vi "qIFC.vi"(0 "System no.":i32=1 min=1 step=1, 2 "Interface parameter":string[](array[string]), 3 "All Parameters?":bool, 5 "error in":errorcluster) -> (14 "Parameter value":string[](array[string]), 15 "interface parameter out":string[](array[string]), 19 "error out":errorcluster)   [LabVIEW 2026]
doc: "Returns the current interface configuration.\n\nE-517, E-518, E-753, E-754, E-871, E-872, E-873, E-874: Note that when the controller is part of a network with DHCP, the static IP address of the controller is returned, not the currently used IP address which was obtained from the DHCP server.\n\nF-206, M-8X0: Only for GCS syntax version = GCS 2.0 or higher (Check with CSV?.vi. If CSV?.vi is not supported, syntax version is GCS 1.0)."
panel:
  # "Returns the current interface configuration."
  # "Query"
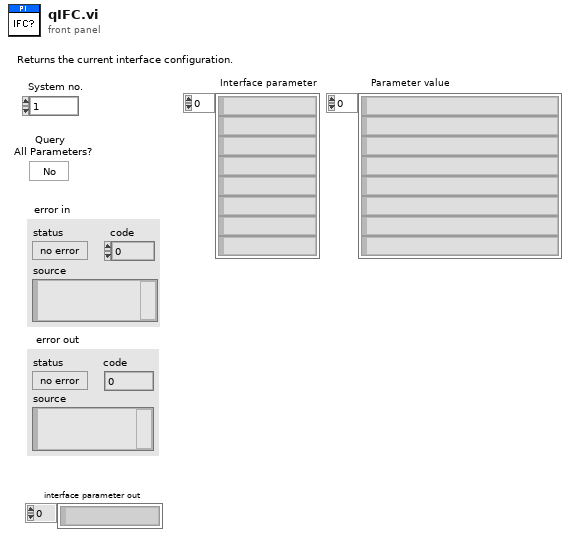
[diagram p1: front panel]
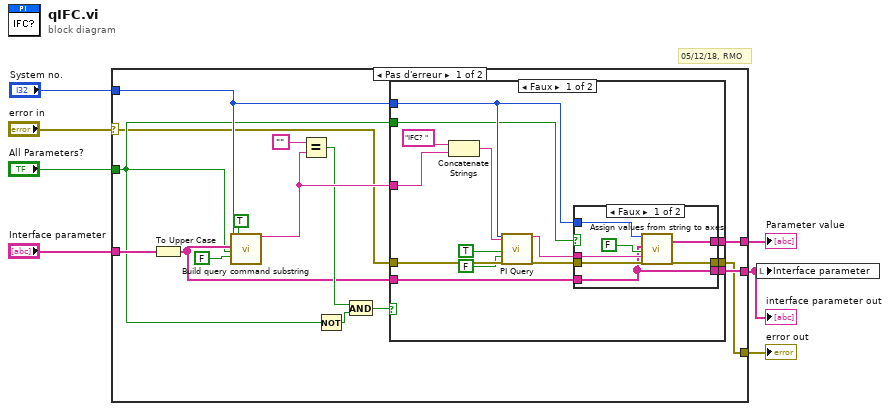
[diagram p0: block diagram]
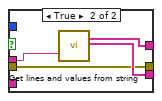
[diagram p2: hidden frame]
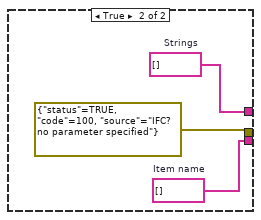
[diagram p3: hidden frame]
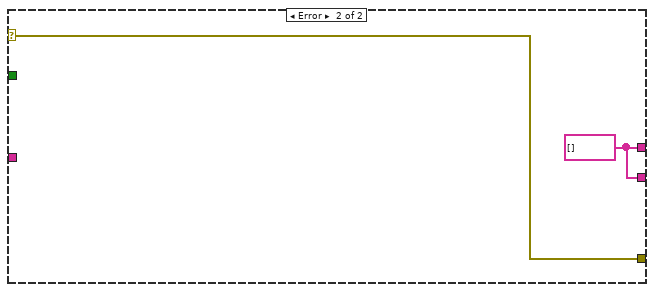
[diagram p4: hidden frame]
diagram:
  # "05/12/18, RMO"
  n1 = case shown="Pas d'erreur" "error in" {
    selector: "error in" -> [w10 w51]
    tunnel: "Interface parameter" -> [w22 _]
    tunnel: [w9 w51] -> w6
    tunnel: "System no." -> [w19 _]
    tunnel: "All Parameters?" -> [w13 _]
    tunnel: [w16 w52] -> w3
    tunnel: [w12 w52] -> w2
    frame No Error {
      n2 = To Upper Case(1:w22) -> (0:w14:string[])
      n3 = call "Build query command substring.vi"("System no."=w19, "Axes to query in"=w14, "Query\nAll axes?"=w13, "For all axes: use\nAxis identifier?"=FALSE ("For all axes: use\nAxis identifier?"), "With space?"=TRUE) -> ("Command substring"=w20:string)  [unwired: 1 in, 13 out]
      n4 = Equal?(x="", y=w20) -> (x = y?=w17:bool)
      n5 = Not(x=w13) -> (.not. x?=w18:bool)
      n6 = And(x=w17, y=w18) -> (x .and. y?=w8:bool)
      n7 = case shown="Faux" w8 {
        tunnel: w20 -> [w33 _]
        tunnel: w19 -> [w32 _]
        tunnel: [w31 w49] -> w16
        tunnel: w14 -> [w30 _]
        tunnel: w13 -> [w29 _]
        tunnel: [w28 w48] -> w12
        tunnel: w10 -> [w27 _]
        tunnel: [w23 errorcluster {"status"=TRUE, "code"=100, "source"="IFC? no parameter specified"} ("error out")] -> w9
        frame False {
          n8 = Concatenate Strings("IFC? ", w33) -> (w34:string)
          n9 = call "PI Query.vi"("System no."=w32, "String to send"=w34, "Attach termination char.?"=TRUE ("Attach Linefeed?"), "Strip spaces?"=FALSE, "error in"=w27) -> ("String read"=w25:string, "error out"=w24:errorcluster)  [unwired: 2 in, 11 out]
          n10 = case shown="Faux" w29 {
            tunnel: w32 -> [w43 _]
            tunnel: w25 -> [w42 w47]
            tunnel: [w41 w46] -> w31
            tunnel: w24 -> [w40 w44]
            tunnel: [w39 w44] -> w23
            tunnel: w30 -> [w37 _]
            tunnel: [w37 w45] -> w28
            frame False {
              n11 = call "Assign values from string to axes.vi"("System no."=w43, "Queried axes"=w37, "All axes queried?"=FALSE, "Input String"=w42, "error in"=w40) -> ("Strings"=w41:string[], "error out"=w39:errorcluster)  [unwired: 4 in, 9 out]
            }
            frame True {
              n12 = call "Get lines and values from string.vi"("Input string"=w47) -> ("Strings"=w46:string[], "Item name"=w45:string[])  [unwired: 1 in, 16 out]
            }
          }
        }
        frame True {
          w48 = string[] []  # Item name
          w49 = string[] []  # Strings
        }
      }
    }
    frame Error {
      w52 = string[] [] ("Strings")
    }
  }
  "error out" <- w6
  "Parameter value" <- w3
  "interface parameter out" <- w2
  n13 = local write "Interface parameter"(w2) -> ()
